vi "Fit Model to Plot Wrapper.vi"(8 "error in (no error)":errorcluster, 11 "Fit Plot Info":T1) -> (0 "error out":errorcluster, 3 "Fit Result String":string)   [LabVIEW 2019]
uses:
  Fit Plot Request Information.ctl
  <vilib>/Utility/miscctls.llb/LVPointDoubleTypeDef.ctl
  Fit Models.ctl
  Fit Settings.ctl
  <vilib>/Analysis/6fits.llb/Curve Fitting Criteria.ctl
  Calc/Ramp Type.ctl
  Residual Type.ctl
  Non-linear Fitting Algorithm.ctl
  <vilib>/Analysis/NI_AALPro.lvlib
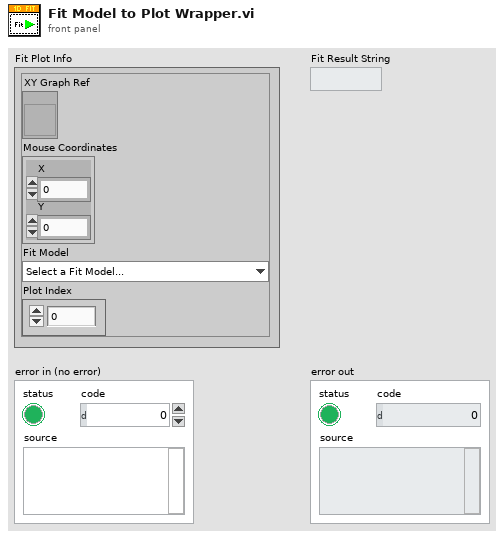
[diagram p1: front panel]
types:
  T1 = typedef "Fit Plot Request Information.ctl" = cluster{"XY Graph Ref":refnum<vi>, "Mouse Coordinates":T2, "Fit Model":T3, "Plot Index":i32}
  T2 = typedef "LVPointDoubleTypeDef.ctl" = cluster{"X":dbl, "Y":dbl}
  T3 = typedef "Fit Models.ctl" = enum16{"Select a Fit Model...", "           Single Peak", "Gaussian", "Asymmetric Gaussian", "Lorentzian", "Asymmetric Lorentzian", "Gaussian/Lorentzian", "Lorentzian/Gaussian", "           Double Peak", "Two Gaussians", "Two Asymmetric Gaussians", "Two H-Connected Gaussians", "Two T-Connected Gaussians", "Two H-Connected Asymmetric Gaussians", "Two T-Connected Asymmetric Gaussians", "           Triple Peak", "Three Gaussians", "Three Asymmetric Gaussians", "              Decays", "1-Exponential", "IRF*PSED", "2-Exponentials", "               ACF", "2D Gaussian ACF", "2D Gaussian + Blinking ACF", "2D Gaussian + Flow ACF", "3D Gaussian ACF", "3D Gaussian + Blinking ACF", "             Multiplot", "2D Gaussian ACF & 2D Gaussian + Flow ACF"}
  T4 = typedef "D-Only Fixed Parameters.ctl" = cluster{"Fix D-only Peak Location":bool, "Peak Location":dbl, "Fix D-only Peak FWHM":bool, "Peak FWHM":dbl}
  T5 = typedef "Fit Settings.ctl" = cluster{"Use Original Plot # Points":bool, "# Fit Plot Points":u32, "Fitting Method":T6, "Weighted Fit":bool, "Show All Fit Components":bool, "Axis Type":T7, "Show Fit Residuals":bool, "Residual Type":T8, "Fitting Algorithm":T9}
  T6 = typedef "NI_AALPro.lvlib/Curve Fitting Criteria.ctl" = u16
  T7 = typedef "Ramp Type.ctl" = u16
  T8 = typedef "Residual Type.ctl" = enum16{"Standard", "Normalized", "Reduced"}
  T9 = typedef "Non-linear Fitting Algorithm.ctl" = enum16{"Levenberg-Marquardt", "Trust-Region Dogleg"}
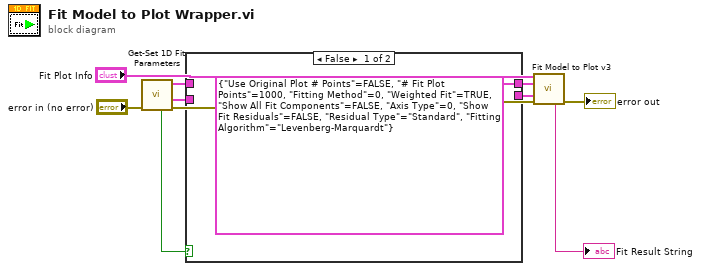
[diagram p0: block diagram]
diagram:
  n1 = call "Get-Set 1D Fit Parameters.vi"("Error In"="error in (no error)") -> ("Error Out"=w5:errorcluster, "Fixed Parameters"=w9:T4, "Fit Settings"=w7:T5, "Initialized?"=w6:bool)  [unwired: 7 in]
  n2 = case shown="False" w6 {
    tunnel: w7 -> [_ w13]
    tunnel: [T5 {"Use Original Plot # Points"=FALSE, "# Fit Plot Points"=1000, "Fitting Method"=0, "Weighted Fit"=TRUE, "Show All Fit Components"=FALSE, "Axis Type"=0, "Show Fit Residuals"=FALSE, "Residual Type"=enum."Standard", "Fitting Algorithm"=enum."Levenberg-Marquardt"} ("Fit Settings") w13] -> w1
    tunnel: [_ w12] -> w8
    tunnel: w9 -> [_ w12]
    frame False {
    }
    frame True {
    }
  }
  n3 = call "Fit Model to Plot v3.vi"("Fit Plot Information"="Fit Plot Info", "Fit Settings"=w1, "Fixed Parameters"=w8, "error in (no error)"=w5) -> ("Fit Result String"=→"Fit Result String":string, "error out"=→"error out":errorcluster)  [unwired: 3 in, 7 out]
